vi "SMBUS Write Word Protocol.vi"(5 "WithPEC":u8, 6 "Data":u16, 7 "CommandCode":u8, 9 "SlaveAddr":i16, 10 "IICIndex":i32, 11 "DevHandle":i32) -> (3 "function return":i32)   [LabVIEW 2010, in "usb2iic.lvlib"]
doc: "int WINAPI SMBUS_WriteWordProtocol(int DevHandle,int IICIndex,short SlaveAddr,unsigned char CommandCode, unsigned short Data,unsigned char WithPEC);"
uses:
  usb2iic.lvlib
  USB2XXX.dll
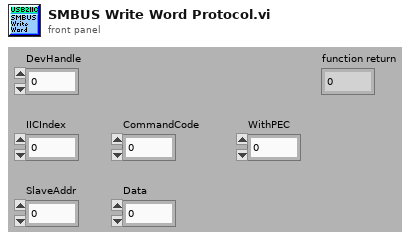
[diagram p1: front panel]
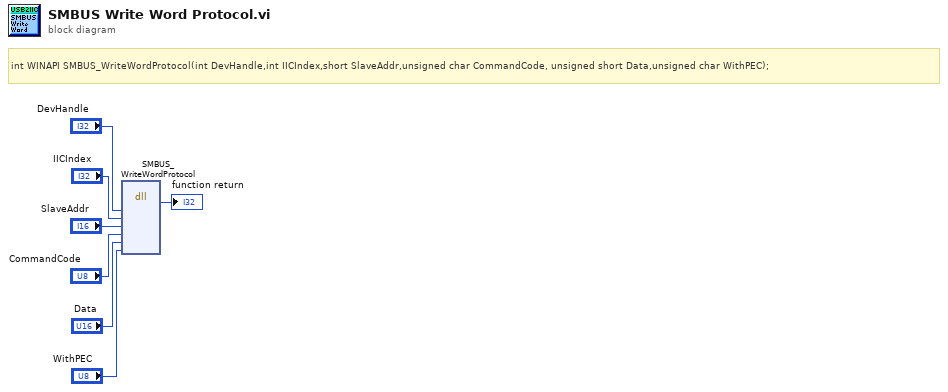
[diagram p0: block diagram]
diagram:
  # "int WINAPI SMBUS_WriteWordProtocol(int DevHandle,int IICIndex,short SlaveAddr,unsigned char CommandCode, unsigned short Data,unsigned char WithPEC);"
  n1 = dll-call lib="G:/OtherWork/USB2XXX_Example/trunk/Labview/PublicFiles/USB2XXX.*" fn="SMBUS_WriteWordProtocol"("DevHandle"="DevHandle", "IICIndex"="IICIndex", "SlaveAddr"="SlaveAddr", "CommandCode"="CommandCode", "Data"="Data", "WithPEC"="WithPEC") -> (→"function return":i32)  [unwired: 9 in, 2 out]
